vi "set_origin.vi"(8 "error in (no error)":errorcluster, 11 "StageDL090602SutterMP285 in":refnum<class "StageDL090602SutterMP285.lvclass">) -> (0 "error out":errorcluster, 3 "StageDL090602SutterMP285 out":refnum<class "StageDL090602SutterMP285.lvclass">)   [LabVIEW 2010, in "StageDL090602SutterMP285.lvclass"]
uses:
  StageDL090602SutterMP285.lvclass
  StageDL090409Scaffold/StageDL090409Scaffold/StageDL090409Scaffold.lvclass
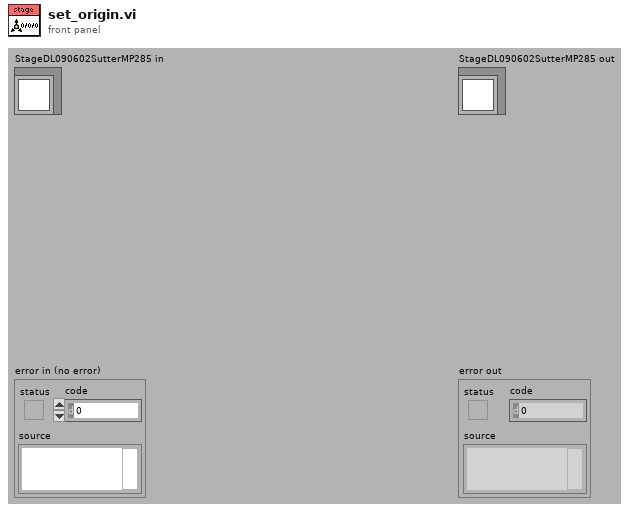
[diagram p1: front panel]
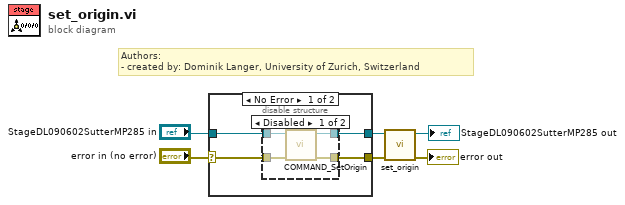
[diagram p0: block diagram]
diagram:
  # "Authors: \n- created by: Dominik Langer, University of Zurich, Switzerland"
  n1 = case shown="No Error" "error in (no error)" {
    selector: "error in (no error)" -> [w7 w17]
    tunnel: [w10 w17] -> w4
    tunnel: [w9 w18] -> w3
    tunnel: "StageDL090602SutterMP285 in" -> [w8 w18]
    frame No Error {
      n2 = disable-structure shown="Disabled" {
        disable-tunnel: [w14 w15] -> w10
        disable-tunnel: [w13 w16] -> w9
        disable-tunnel: w8 -> [w12 w16]
        disable-tunnel: w7 -> [w11 w15]
        frame Disabled {
          n3 = call-dynamic "COMMAND_SetOrigin.vi"("error in (no error)"=w11, "StageDL090602SutterMP285 in"=w12) -> ("error out"=w14:errorcluster, "StageDL090602SutterMP285 out"=w13:refnum<class "StageDL090602SutterMP285.lvclass">)  [unwired: 8 in]
        }
        frame Enabled {
        }
      }
    }
    frame Error {
    }
  }
  n4 = call-parent "set_origin.vi"("error in (no error)"=w4, "StageDL090409Scaffold in"=w3) -> ("error out"=→"error out":errorcluster, "StageDL090409Scaffold out"=→"StageDL090602SutterMP285 out":refnum<class "StageDL090602SutterMP285.lvclass">)  [unwired: 8 in]
